vi "TestMode_Operation_SUB_VI_default.vi"(6 "error in (no error)":errorcluster, 7 "Response ID 1":u8=68, 8 "Operation Message Length 1":i32, 9 "Operation Message ID 1":i32=67, 10 "Socket Port":u16=1600, 11 "Socket IP Adress":string="192.168.1.100") -> (1 "End frequency and Time Stamp 2":string, 3 "error out":errorcluster)   [LabVIEW 2017]
panel:
  out "connection ID out":refnum<k5>
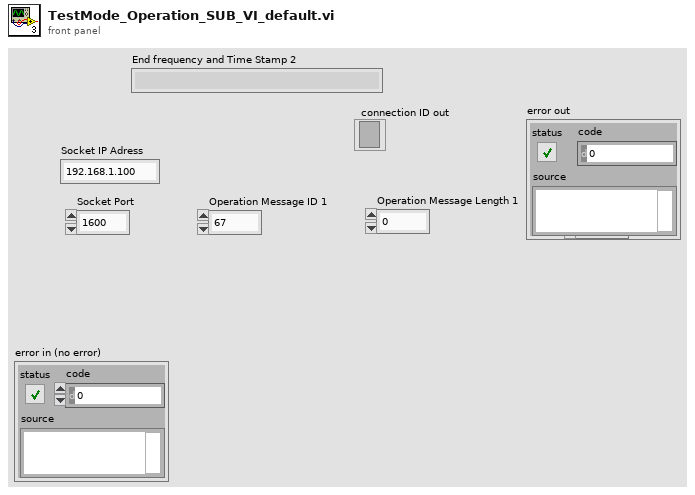
[diagram p1: front panel]
types:
  T1 = cluster{"Seek Request Message Length to DB ":i32, "Seek Request Message ID to DB":i32}
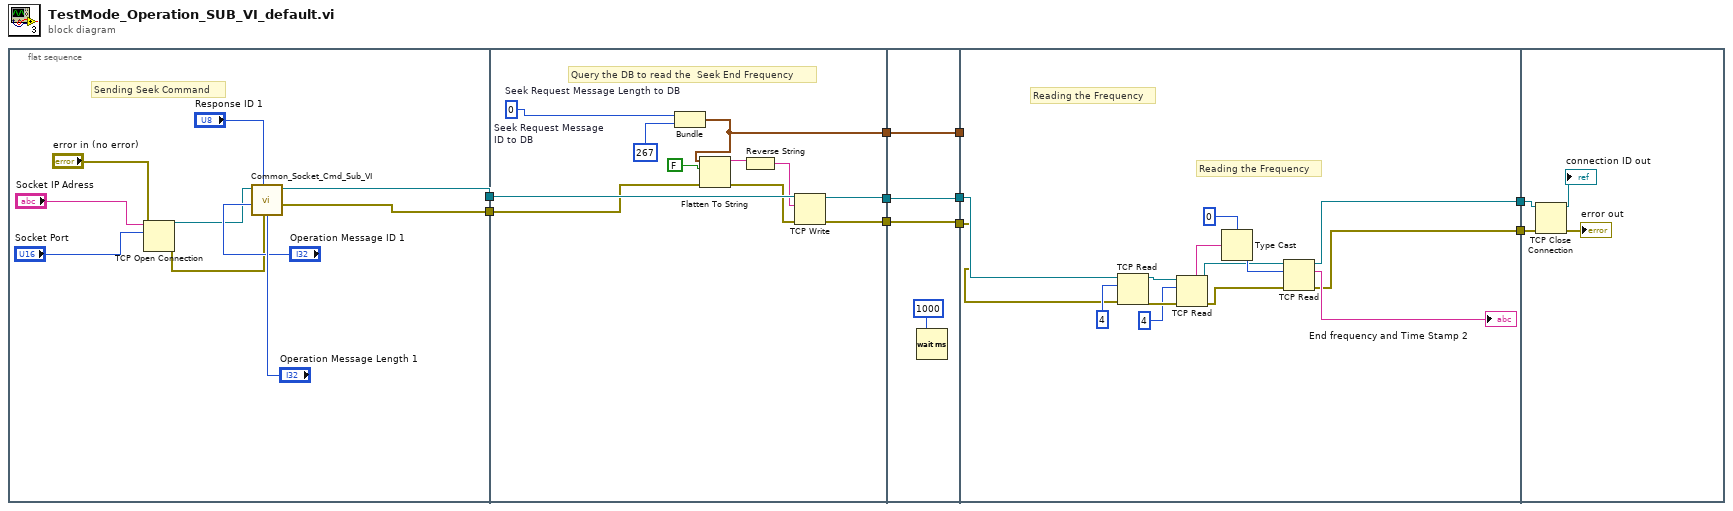
[diagram p0: block diagram]
diagram:
  n1 = flat-sequence {
    tunnel: [w20] -> w10
    tunnel: [w19] -> w3
    tunnel: w10 -> [w31]
    tunnel: [w24] -> w9
    tunnel: [w23] -> w8
    tunnel: [w22] -> w7
    tunnel: w3 -> [w27]
    tunnel: w9 -> [w33]
    tunnel: w8 -> [w34]
    tunnel: [w34] -> w6
    tunnel: [w33] -> w5
    tunnel: [w32] -> w4
    tunnel: w7 -> [w32]
    tunnel: [w39] -> w2
    tunnel: [w38] -> w1
    tunnel: w6 -> [w37]
    tunnel: w5 -> [w36]
    tunnel: w4 -> [_]
    tunnel: w2 -> [w51]
    tunnel: w1 -> [w50]
    frame #0 {
      # "Sending Seek Command"
      n2 = TCP Open Connection(address="Socket IP Adress", remote port or service name="Socket Port", error in (no error)="error in (no error)") -> (connection ID=w13:refnum<k5>, error out=w14:errorcluster)  [unwired: 2 in]
      n3 = call "Common_Socket_Cmd_Sub_VI.vi"("Common Socket Error in"=w14, "Response ID 1"="Response ID 1", "Operation Message Length 1"="Operation Message Length 1", "Operation Message ID 1"="Operation Message ID 1", "connection ID"=w13) -> ("error out"=w19:errorcluster, "connection ID"=w20:refnum<k5>)  [unwired: 4 in, 1 out]
    }
    frame #1 {
      w29 = 267  # Seek Request Message ID to DB
      w30 = 0  # Seek Request Message Length to DB
      # "Query the DB to read the  Seek End Frequency"
      n4 = Bundle("Seek Request Message Length to DB"=w30, "Seek Request Message ID to DB"=w29) -> (w22:T1)  [unwired: 1 in]
      n5 = Flatten To String(anything=w22, prepend array or string size? (T)=FALSE, error in (no error)=w27) -> (data string=w28:string, error out=w25:errorcluster)  [unwired: 1 in, 1 out]
      n6 = Reverse String(1:w28) -> (0:w26:string)
      n7 = TCP Write(connection ID=w31, data in=w26, error in (no error)=w25) -> (connection ID out=w23:refnum<k5>, error out=w24:errorcluster)  [unwired: 1 in, 1 out]
    }
    frame #2 {
      n8 = Wait (ms)(milliseconds to wait=u32 1000) -> ()  [unwired: 1 out]
    }
    frame #3 {
      # "Reading the Frequency"
      # "Reading the Frequency"
      n9 = TCP Read(connection ID=w37, bytes to read=4, error in (no error)=w36) -> (connection ID out=w48:refnum<k5>, error out=w47:errorcluster)  [unwired: 2 in, 1 out]
      n10 = TCP Read(connection ID=w48, bytes to read=4, error in (no error)=w47) -> (connection ID out=w42:refnum<k5>, data out=w45:string, error out=w41:errorcluster)  [unwired: 2 in]
      n11 = Type Cast(type=u8 0 ("bytes to read"), x=w45) -> (*(type *) &x=w43:u8)
      n12 = TCP Read(connection ID=w42, bytes to read=w43, error in (no error)=w41) -> (connection ID out=w39:refnum<k5>, data out=→"End frequency and Time Stamp 2":string, error out=w38:errorcluster)  [unwired: 2 in]
    }
    frame #4 {
      n13 = TCP Close Connection(connection ID=w51, error in (no error)=w50) -> (connection ID out=→"connection ID out":refnum<k5>, error out=→"error out":errorcluster)  [unwired: 1 in]
    }
  }
